vi "New Rotating Daily File Sink.vi"(8 "error in (no error)":errorcluster, 11 "File Path":path) -> (0 "error out":errorcluster, 3 "Rotating Daily File Sink out":refnum<class "Rotating Daily File Sink.lvclass">)   [LabVIEW 2020, in "LV Log.lvlib" / "Rotating Daily File Sink.lvclass"]
uses:
  Rotating Daily File Sink.lvclass
  Rotating Daily File Sink.lvclass/Rotating Daily File Sink.ctl
  File Sink/File Sink.lvclass
  C:/Users/hughe_cx/Documents/05_repos/LVLog/Source/Sinks/File Sink/File Sink.lvclass
  C:/Users/hughe_cx/Documents/05_repos/LVLog/Source/Sinks/Sink/Sink.lvclass
  C:/Users/hughe_cx/Documents/05_repos/LVLog/Source/Sinks/Rotating File Sink/Rotating Daily File Sink.lvclass
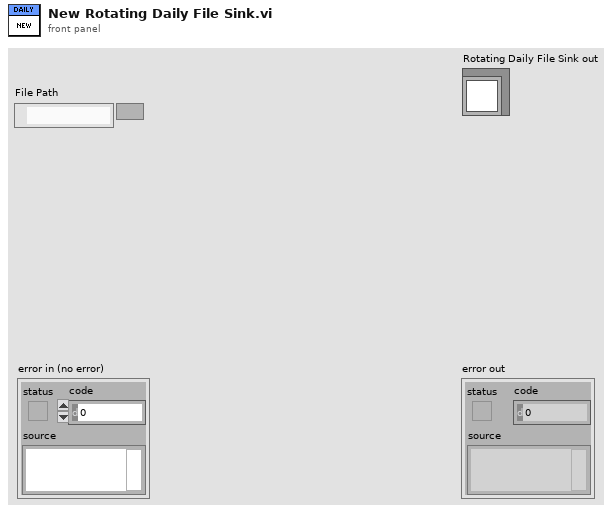
[diagram p1: front panel]
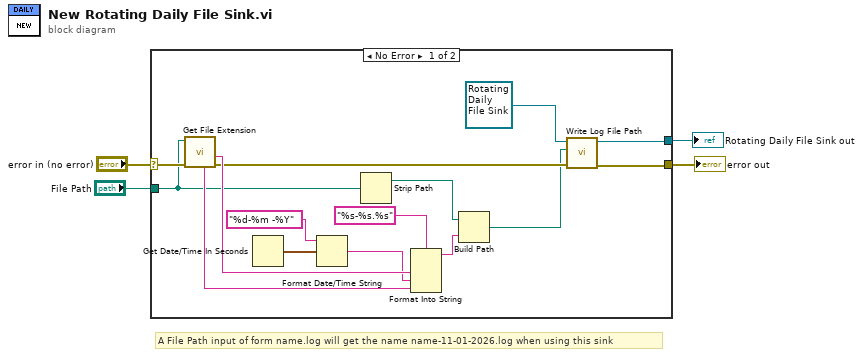
[diagram p0: block diagram]
diagram:
  # "A File Path input of form name.log will get the name name-11-01-2026.log when using this sink"
  n1 = case shown="No Error" "error in (no error)" {
    selector: "error in (no error)" -> [w19 w20]
    tunnel: [w5 w20] -> w4
    tunnel: [w6 _] -> w3
    tunnel: "File Path" -> [w15 _]
    frame No Error {
      n2 = call <vilib>:"Get File Extension.vi"("error in (no error)"=w19, "file"=w15) -> ("error out"=w8:errorcluster, "filename without extension"=w17:string, "unmodified file extension"=w16:string)  [unwired: 5 in, 2 out]
      n3 = Get Date/Time In Seconds() -> (seconds since 1Jan1904=w12:timestamp)
      n4 = Format Date/Time String(time format string (%c)="%d-%m -%Y", seconds (now)=w12) -> (date/time string=w11:string)  [unwired: 1 in]
      n5 = Strip Path(path=w15) -> (stripped path=w14:path)  [unwired: 1 out]
      n6 = Format Into String(format string="%s-%s.%s", w17, w11, w16) -> (resulting string=w13:string)  [unwired: 2 in, 1 out]
      n7 = Build Path(base path=w14, name or relative path=w13) -> (appended path=w7:path)
      n8 = call "Write Log File Path.vi"("error in (no error)"=w8, "Log File Path"=w7, "File Sink in"=refnum<class "Rotating Daily File Sink.lvclass"> refnum ("Rotating Daily File Sink out")) -> ("error out"=w5:errorcluster, "File Sink out"=w6:refnum<class "Rotating Daily File Sink.lvclass">)  [unwired: 7 in]
    }
    frame Error {
    }
  }
  "error out" <- w4
  "Rotating Daily File Sink out" <- w3
